vi "For_Loop.vi"() -> ()   [LabVIEW 2015]
panel:
  out "XY Graph":cluster{"X":dbl, "Y":dbl}[](graph)=[{"X"=0.0, "Y"=0.0}, {"X"=3.420201433256687, "Y"=2.7563735581699915}, {"X"=6.4278760968653925, "Y"=5.299192642332049}, {"X"=8.660254037844386, "Y"=7.431448254773941}, {"X"=9.84807753012208, "Y"=8.98794046299167}, {"X"=9.84807753012208, "Y"=9.848077530122081}, {"X"=8.660254037844387, "Y"=9.945218953682733}, {"X"=6.427876096865395, "Y"=9.271838545667874}, {"X"=3.420201433256689, "Y"=7.88010753606722}, {"X"=1.2246467991473533e-15, "Y"=5.877852522924733}, {"X"=-3.4202014332566866, "Y"=3.420201433256685}, {"X"=-6.427876096865389, "Y"=0.6975647374412508}, {"X"=-8.660254037844384, "Y"=-2.079116908177591}, {"X"=-9.84807753012208, "Y"=-4.694715627858908}, {"X"=-9.848077530122081, "Y"=-6.9465837045899725}, {"X"=-8.66025403784439, "Y"=-8.660254037844389}, {"X"=-6.427876096865396, "Y"=-9.702957262759965}, {"X"=-3.420201433256694, "Y"=-9.993908270190957}, {"X"=-2.4492935982947065e-15, "Y"=-9.510565162951536}, {"X"=3.4202014332566892, "Y"=-8.290375725550415}, {"X"=6.4278760968653925, "Y"=-6.427876096865389}, {"X"=8.660254037844378, "Y"=-4.0673664307580015}, {"X"=9.84807753012208, "Y"=-1.3917310096006499}, {"X"=9.848077530122081, "Y"=1.3917310096006628}, {"X"=8.66025403784439, "Y"=4.067366430757997}, {"X"=6.427876096865404, "Y"=6.4278760968653925}, {"X"=3.420201433256687, "Y"=8.290375725550419}, {"X"=3.673940397442059e-15, "Y"=9.510565162951535}, {"X"=-3.42020143325668, "Y"=9.993908270190957}, {"X"=-6.4278760968653845, "Y"=9.702957262759963}, {"X"=-8.660254037844378, "Y"=8.660254037844382}, {"X"=-9.848077530122076, "Y"=6.946583704589977}, {"X"=-9.848077530122081, "Y"=4.694715627858909}, {"X"=-8.66025403784439, "Y"=2.0791169081775913}, {"X"=-6.427876096865405, "Y"=-0.6975647374412415}, {"X"=-3.4202014332566884, "Y"=-3.42020143325668}, {"X"=-4.898587196589413e-15, "Y"=-5.877852522924728}, {"X"=3.420201433256679, "Y"=-7.88010753606722}, {"X"=6.427876096865397, "Y"=-9.271838545667876}, {"X"=8.660254037844378, "Y"=-9.945218953682733}, {"X"=9.84807753012208, "Y"=-9.84807753012208}, {"X"=9.848077530122083, "Y"=-8.987940462991672}, {"X"=8.660254037844402, "Y"=-7.431448254773941}, {"X"=6.427876096865406, "Y"=-5.299192642332045}, {"X"=3.420201433256706, "Y"=-2.756373558169983}, {"X"=6.123233995736766e-15, "Y"=-4.898587196589413e-15}, {"X"=-3.4202014332566777, "Y"=2.756373558170008}, {"X"=-6.427876096865383, "Y"=5.299192642332052}, {"X"=-8.660254037844377, "Y"=7.431448254773935}, {"X"=-9.848077530122076, "Y"=8.987940462991675}, {"X"=-9.848077530122085, "Y"=9.84807753012208}, {"X"=-8.660254037844402, "Y"=9.945218953682735}, {"X"=-6.4278760968653925, "Y"=9.271838545667872}, {"X"=-3.420201433256724, "Y"=7.880107536067226}, {"X"=-7.347880794884118e-15, "Y"=5.877852522924735}, {"X"=3.4202014332566764, "Y"=3.4202014332566892}, {"X"=6.427876096865381, "Y"=0.6975647374412512}, {"X"=8.660254037844377, "Y"=-2.0791169081775815}, {"X"=9.848077530122076, "Y"=-4.694715627858916}, {"X"=9.848077530122087, "Y"=-6.9465837045899566}, {"X"=8.660254037844403, "Y"=-8.660254037844394}, {"X"=6.427876096865393, "Y"=-9.702957262759961}, {"X"=3.4202014332567248, "Y"=-9.993908270190957}, {"X"=8.572527594031473e-15, "Y"=-9.510565162951538}, {"X"=-3.4202014332566755, "Y"=-8.290375725550419}, {"X"=-6.42787609686538, "Y"=-6.4278760968653925}, {"X"=-8.660254037844377, "Y"=-4.067366430757998}, {"X"=-9.848077530122076, "Y"=-1.391731009600646}, {"X"=-9.848077530122087, "Y"=1.3917310096006315}, {"X"=-8.660254037844403, "Y"=4.0673664307580175}, {"X"=-6.427876096865395, "Y"=6.427876096865381}, {"X"=-3.420201433256726, "Y"=8.290375725550431}, {"X"=-9.797174393178826e-15, "Y"=9.510565162951533}, {"X"=3.4202014332566746, "Y"=9.993908270190957}, {"X"=6.427876096865379, "Y"=9.702957262759965}, {"X"=8.660254037844357, "Y"=8.660254037844386}, {"X"=9.848077530122083, "Y"=6.946583704589968}, {"X"=9.848077530122087, "Y"=4.694715627858898}, {"X"=8.660254037844403, "Y"=2.0791169081775784}, {"X"=6.427876096865423, "Y"=-0.6975647374412365}, {"X"=3.4202014332566937, "Y"=-3.420201433256709}, {"X"=1.1021821192326179e-14, "Y"=-5.877852522924724}, {"X"=-3.4202014332566733, "Y"=-7.880107536067217}, {"X"=-6.427876096865379, "Y"=-9.271838545667872}, {"X"=-8.660254037844357, "Y"=-9.945218953682733}, {"X"=-9.848077530122083, "Y"=-9.84807753012208}, {"X"=-9.848077530122087, "Y"=-8.987940462991666}, {"X"=-8.660254037844403, "Y"=-7.431448254773957}, {"X"=-6.427876096865424, "Y"=-5.299192642332034}, {"X"=-3.4202014332567283, "Y"=-2.756373558170005}, {"X"=-1.2246467991473532e-14, "Y"=-9.797174393178826e-15}, {"X"=3.420201433256672, "Y"=2.756373558169986}, {"X"=6.427876096865378, "Y"=5.299192642332078}, {"X"=8.660254037844373, "Y"=7.431448254773944}, {"X"=9.848077530122076, "Y"=8.987940462991673}, {"X"=9.848077530122087, "Y"=9.848077530122083}, {"X"=8.660254037844405, "Y"=9.945218953682737}, {"X"=6.4278760968654245, "Y"=9.271838545667881}, {"X"=3.420201433256729, "Y"=7.880107536067207}, {"X"=4.899825157862589e-14, "Y"=5.877852522924711}]
  in  "Amplitude 2":dbl=10.0
  in  "Phase 2":dbl
  in  "Frequency 2":dbl=50.0
  in  "Sampling Frequency 2":dbl=900.0
  in  "Number of Cycles 2":i32=100
  in  "Amplitude":dbl=10.0
  in  "Phase":dbl
  in  "Frequency":dbl=40.0
  in  "Sampling Frequency":dbl=900.0
  in  "Number of Cycles":i32=100
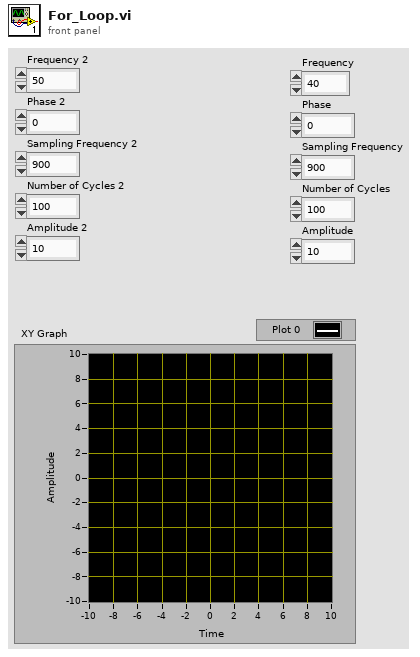
[diagram p1: front panel]
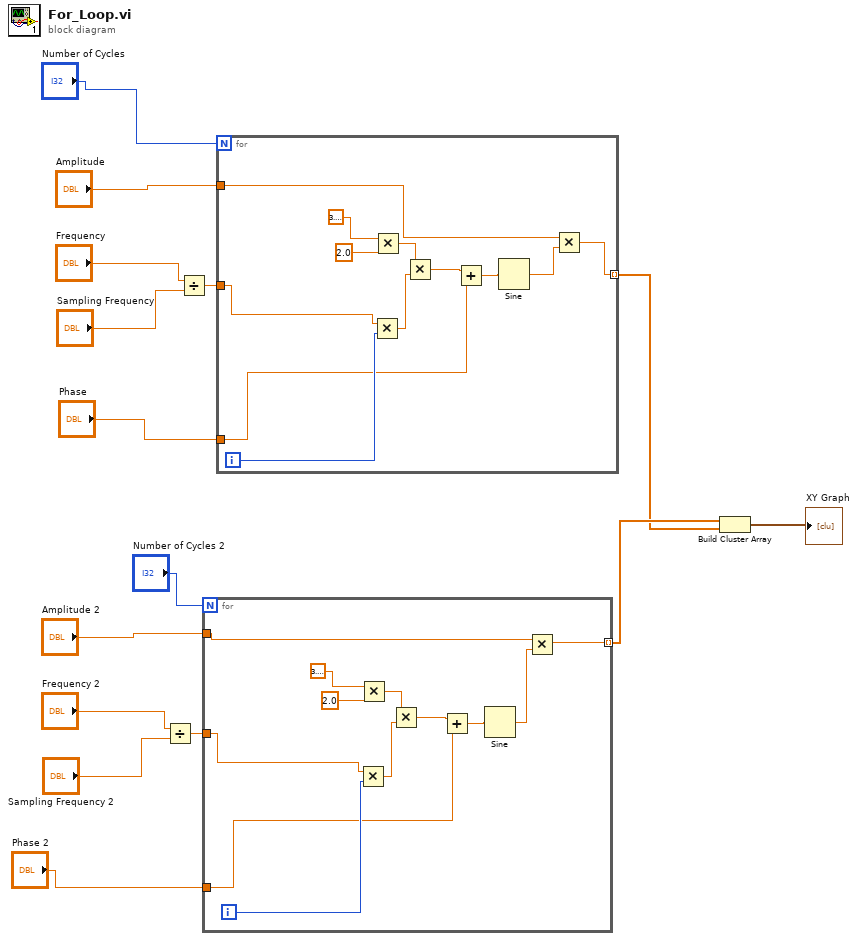
[diagram p0: block diagram]
diagram:
  n1 = Divide(x="Frequency 2", y="Sampling Frequency 2") -> (x/y=w6:dbl)
  n2 = Divide(x="Frequency", y="Sampling Frequency") -> (x/y=w11:dbl)
  n3 = for {
    N: "Number of Cycles 2" -> [_]
    tunnel: [w20] -> w3 mode=indexing
    tunnel: "Phase 2" -> [w21]
    tunnel: "Amplitude 2" -> [w18]
    tunnel: w6 -> [w17]
    i -> [w25]
    n4 = Multiply(x=w17, y=w25) -> (x*y=w24:dbl)
    n5 = Multiply(x=3.141592653589793, y=2.0) -> (x*y=w27:dbl)
    n6 = Multiply(x=w27, y=w24) -> (x*y=w23:dbl)
    n7 = Add(x=w23, y=w21) -> (x+y=w22:dbl)
    n8 = Sine(x=w22) -> (sin(x)=w19:dbl)
    n9 = Multiply(x=w18, y=w19) -> (x*y=w20:dbl)
  }
  n10 = for {
    N: "Number of Cycles" -> [_]
    tunnel: [w32] -> w2 mode=indexing
    tunnel: "Phase" -> [w33]
    tunnel: "Amplitude" -> [w30]
    tunnel: w11 -> [w29]
    i -> [w37]
    n11 = Multiply(x=w29, y=w37) -> (x*y=w36:dbl)
    n12 = Multiply(x=3.141592653589793, y=2.0) -> (x*y=w39:dbl)
    n13 = Multiply(x=w39, y=w36) -> (x*y=w35:dbl)
    n14 = Add(x=w35, y=w33) -> (x+y=w34:dbl)
    n15 = Sine(x=w34) -> (sin(x)=w31:dbl)
    n16 = Multiply(x=w30, y=w31) -> (x*y=w32:dbl)
  }
  n17 = Build Cluster Array(w3, w2) -> (→"XY Graph":cluster{dbl, dbl}[])
